vi "Main Tclk.vi"() -> ()   [LabVIEW 2018] (continued)
                        n3304 = call <vilib>:"Flatten Pixmap.vi"("colors"=u32[] [16777222, 65793, 131586, 197379, 263172, 328965, 394758, 460551, 526344, 592137, 657930, 723723, 789516, 855309, 921102, 986895, 1052688, 1118481, 1184274, 1250067, 1315860, 1381653, 1447446, 1513239, 1579032, 1644825, 1710618, 1776411, 1842204, 1907997, 1973790, 2039583, 2105376, 2171169, 2236962, 2302755, 2368548, 2434341, 2500134, 2565927, 2631720, 2697513, 2763306, 2829099, 2894892, 2960685, 3026478, 3092271, 3158064, 3223857, 3289650, 3355443, 3421236, 3487029, 3552822, 3618615, 3684408, 3750201, 3815994, 3881787, 3947580, 4013373, 4079166, 4144959, 4210752, 4276545, 4342338, 4408131, 4473924, 4539717, 4605510, 4671303, 4737096, 4802889, 4868682, 4934475, 5000268, 5066061, 5131854, 5197647, 5263440, 5329233, 5395026, 5460819, 5526612, 5592405, 5658198, 5723991, 5789784, 5855577, 5921370, 5987163, 6052956, 6118749, 6184542, 6250335, 6316128, 6381921, 6447714, 6513507, 6579300, 6645093, 6710886, 6776679, 6842472, 6908265, 6974058, 7039851, 7105644, 7171437, 7237230, 7303023, 7368816, 7434609, 7500402, 7566195, 7631988, 7697781, 7763574, 7829367, 7895160, 7960953, 8026746, 8092539, 8158332, 8224125, 8289918, 8355711, 8421504, 8487297, 8553090, 8618883, 8684676, 8750469, 8816262, 8882055, 8947848, 9013641, 9079434, 9145227, 9211020, 9276813, 9342606, 9408399, 9474192, 9539985, 9605778, 9671571, 9737364, 9803157, 9868950, 9934743, 10000536, 10066329, 10132122, 10197915, 10263708, 10329501, 10395294, 10461087, 10526880, 10592673, 10658466, 10724259, 10790052, 10855845, 10921638, 10987431, 11053224, 11119017, 11184810, 11250603, 11316396, 11382189, 11447982, 11513775, 11579568, 11645361, 11711154, 11776947, 11842740, 11908533, 11974326, 12040119, 12105912, 12171705, 12237498, 12303291, 12369084, 12434877, 12500670, 12566463, 12632256, 12698049, 12763842, 12829635, 12895428, 12961221, 13027014, 13092807, 13158600, 13224393, 13290186, 13355979, 13421772, 13487565, 13553358, 13619151, 13684944, 13750737, 13816530, 13882323, 13948116, 14013909, 14079702, 14145495, 14211288, 14277081, 14342874, 14408667, 14474460, 14540253, 14606046, 14671839, 14737632, 14803425, 14869218, 14935011, 15000804, 15066597, 15132390, 15198183, 15263976, 15329769, 15395562, 15461355, 15527148, 15592941, 15658734, 15724527, 15790320, 15856113, 15921906, 15987699, 16053492, 16119285, 16185078, 16250871, 16316664, 16382457, 16448250, 16514043, 16579836, 16645629, 16711422, 16448250] ("256 gray scale"), "8-bit pixmap"=w9681) -> ("image data"=w9684:T52)  [unwired: 4 in, 5 out]
                        n3305 = call <vilib>:"Write PNG File.vi"("image data"=w9684, "path to PNG file"=w9685) -> ()  [unwired: 1 in, 9 out]
                      }
                    }
                  }
                }
                n3306 = Open/Create/Replace File(file path (use dialog)=w9608) -> (error out=w9610:errorcluster)  [unwired: 5 in, 2 out]
                n3307 = Unbundle By Name(w9610) -> ("status"=w9609:bool)
                n3308 = local read "Recipe input"() -> (w9606:T7)
                n3309 = case shown="False" w9609 {
                  tunnel: w9608 -> [w9663 w9664]
                  tunnel: [w9662 w9664] -> w9611
                  frame False {
                    n3310 = Delete(path (use dialog)=w9663) -> (deleted path=w9662:path)  [unwired: 4 in, 2 out]
                  }
                  frame True {
                  }
                }
                n3311 = call "Recipe read write.vi"("Write"=TRUE, "Recipe path"=w9611, "Write input"=w9606) -> ()  [unwired: 5 in, 4 out]
                n3312 = local read "FIB"() -> (w9602:bool)
                n3313 = Greater Than 0?(x="SEM-FIB Delay (s)") -> (x > 0?=w9600:bool)
                n3314 = Compound Arithmetic op=AND(w9600, "After SEM", w9602) -> (w9604:bool)
                n3315 = case shown="True" w9604 {
                  tunnel: "SEM-FIB Delay (s)" -> [_ w9622]
                  frame False {
                  }
                  frame True {
                    n3316 = local read "FIB blank condenser %"() -> (w9631:u8)
                    n3317 = Number To Decimal String(number=w9622) -> (decimal integer string=w9626:string)  [unwired: 1 in]
                    n3318 = expression code="x*10"(w9622) -> (w9623:u32)
                    n3319 = for {
                      N: w9623 -> [_]
                      stop <- w9634 stop-if-true
                      n3320 = local read "Mill Manual Pause"() -> (w9635:bool)
                      n3321 = local read "FIB"() -> (w9637:bool)
                      n3322 = Wait Until Next ms Multiple(millisecond multiple=u32 100) -> ()  [unwired: 1 out]
                      n3323 = Not(x=w9637) -> (.not. x?=w9636:bool)
                      n3324 = Or(x=w9636, y=w9635) -> (x .or. y?=w9634:bool)
                    }
                    n3325 = Concatenate Strings(w9626, " s delay after SEM..." ("string")) -> (w9624:string)
                    n3326 = Less?(x=w9631, y=u8 100) -> (x < y?=w9633:bool)
                    n3327 = Greater Or Equal?(x=w9622, y=5.0) -> (x >= y?=w9632:bool)
                    n3328 = local write "Status message"(w9624) -> ()
                    n3329 = To Single Precision Float(number=w9631) -> (single precision float=w9630:sgl)
                    n3330 = Compound Arithmetic op=AND(w9633, w9632) -> (w9629:bool)
                    n3331 = case shown="True" w9629 {
                      tunnel: w9630 -> [_ w9640]
                      tunnel: w9622 -> [_ w9639]
                      frame False {
                      }
                      frame True {
                        n3332 = stacked-sequence {
                          seq-local: [w9642 _ _ _] -> [_ w9650 _ _]
                          seq-local: [w9641 _ _ _] -> [_ w9648 _ w9659]
                          seq-local: [_ w9649 _ _] -> [_ _ _ w9660]
                          tunnel: w9640 -> [_ w9647 _ _]
                          tunnel: w9639 -> [_ _ w9653 _]
                          frame #0 {
                            n3333 = local read "Api"() -> (w9644:refnum<k7>)
                            n3334 = call "SmartSEM Remote API get float.vi"("lpszParam"="AP_FIB_CONDENSER" ("Status message"), "ActiveX Container"=w9644) -> ("vValue"=w9641:sgl, "reference out"=w9642:refnum<k7>)  [unwired: 7 in, 1 out]
                          }
                          frame #1 {
                            n3335 = Compound Arithmetic op=MULTIPLY(w9648, w9647, sgl 0.01 ("value")) -> (w9646:sgl)
                            n3336 = call "SmartSEM Remote API set float.vi"("vValue"=w9646, "lpszParam"="AP_FIB_CONDENSER" ("Status message"), "ActiveX Container"=w9650) -> ("reference out"=w9649:refnum<k7>)  [unwired: 7 in, 1 out]
                          }
                          frame #2 {
                            n3337 = expression code="(x-3)*10"(w9653) -> (w9652:u32)
                            n3338 = for {
                              N: w9652 -> [_]
                              stop <- w9654 stop-if-true
                              n3339 = local read "Mill Manual Pause"() -> (w9655:bool)
                              n3340 = local read "FIB"() -> (w9657:bool)
                              n3341 = Wait Until Next ms Multiple(millisecond multiple=u32 100) -> ()  [unwired: 1 out]
                              n3342 = Not(x=w9657) -> (.not. x?=w9656:bool)
                              n3343 = Or(x=w9656, y=w9655) -> (x .or. y?=w9654:bool)
                            }
                          }
                          frame #3 {
                            n3344 = call "SmartSEM Remote API set float.vi"("vValue"=w9659, "lpszParam"="AP_FIB_CONDENSER" ("Status message"), "ActiveX Container"=w9660) -> ()  [unwired: 7 in, 2 out]
                          }
                        }
                      }
                    }
                  }
                }
              }
              frame #40 {
                n3345 = local read "Milling para"() -> (w9706:T35)
                n3346 = local read "SEM Scan Parameters"() -> (w9726:T26)
                n3347 = local read "Temp array"() -> (w9787:sgl[])
                n3348 = local read "Alert Settings"() -> (w9780:T36)
                n3349 = Unbundle By Name(w9706) -> ("FIB PID target"=w9761:sgl, "FIB PID on"=w9766:bool, "FIB PID measured"=w9764:u8)
                n3350 = Unbundle By Name(w9726) -> ("Pixel size (nm)"=w9721:sgl)
                n3351 = Unbundle By Name(w9706) -> ("FIB PID on"=w9728:bool, "FIB PID measured"=w9727:u8, "Lines auto pause"=w9767:u16)
                n3352 = Unbundle By Name(w9780) -> ("Focus index warning"=w9785:bool)
                n3353 = Unbundle By Name(w9706) -> ("Z-step (nm)"=w9768:dbl)
                n3354 = local read "FI below limit counts"() -> (w9786:u8)
                n3355 = Unbundle By Name(w9780) -> ("Focus index stop limit"=w9783:sgl)
                n3356 = Unbundle By Name(w9780) -> ("Temp limit auto"=w9790:bool)
                n3357 = local read "Focus Index"() -> (w9770:sgl)
                n3358 = Array Size(array=w9787) -> (size(s)=w9791:i32)
                n3359 = Equal?(x=u8 3, y=w9764) -> (x = y?=w9765:bool)
                n3360 = In Range and Coerce(upper limit=sgl 50.0, x=w9721, lower limit=sgl 8.0) -> (coerced(x)=w9722:sgl)  [unwired: 1 out]
                n3361 = Greater Or Equal?(x=w9791, y=10 ("x")) -> (x >= y?=w9789:bool)
                n3362 = And(x=w9766, y=w9765) -> (x .and. y?=w9762:bool)
                n3363 = And(x=w9789, y=w9790) -> (x .and. y?=w9788:bool)
                n3364 = Multiply(x=w9767, y=w9768) -> (x*y=w9725:dbl)
                n3365 = case shown="True" w9762 {
                  tunnel: w9761 -> [_ w9805]
                  tunnel: [FALSE w9804] -> w9760
                  frame False {
                  }
                  frame True {
                    n3366 = local read "Faraday Cup (nA)"() -> (w9806:sgl)
                    n3367 = Greater?(x=w9805, y=w9806) -> (0:w9804:bool)
                  }
                }
                "Faraday Cup < Milling current" <- w9760
                n3368 = case shown="True" w9788 {
                  tunnel: w9787 -> [_ w9843]
                  tunnel: w9780 -> [w9837 w9844]
                  tunnel: [w9837 w9838] -> _
                  frame False {
                  }
                  frame True {
                    n3369 = call "Auto limits.vi"("Minimum half range"=0.8, "# of interquartile range or stdev"=4.0 ("# of sigma"), "Input array"=w9843) -> ("Low limit"=w9841:dbl, "High limit"=w9842:dbl)  [unwired: 6 in, 1 out]
                    n3370 = Bundle By Name(cluster=w9844, "High limit (F)"=w9842, "Low limit (F)"=w9841) -> (w9838:T36)
                    n3371 = local write "Alert Settings"(w9838) -> ()
                  }
                }
                n3372 = Divide(x=w9722, y=w9725) -> (x/y=w9707:dbl)
                n3373 = Greater Or Equal?(x=w9770, y=w9783) -> (x >= y?=w9784:bool)
                n3374 = case shown="True" w9728 {
                  tunnel: [FALSE w9809] -> w9777
                  tunnel: w9727 -> [_ w9808]
                  frame False {
                  }
                  frame True {
                    n3375 = case shown="3" w9808 {
                      tunnel: [w9811 w9816 w9820 w9827 FALSE] -> w9809
                      frame 0 {
                        n3376 = local read "Specimen I out of bound"() -> (w9814:bool)
                        n3377 = local read "BD1 out of bound"() -> (w9810:bool)
                        n3378 = local read "BD2 out of bound"() -> (w9813:bool)
                        n3379 = local read "Milling I out of bound"() -> (w9812:bool)
                        n3380 = Compound Arithmetic op=OR(w9814, w9810, w9813, w9812) -> (w9811:bool)
                      }
                      frame 1 {
                        n3381 = local read "Specimen I out of bound"() -> (w9818:bool)
                        n3382 = local read "BD1 out of bound"() -> (w9815:bool)
                        n3383 = local read "BD2 out of bound"() -> (w9817:bool)
                        n3384 = Compound Arithmetic op=OR(w9818, w9815, w9817) -> (w9816:bool)
                      }
                      frame 2 {
                        n3385 = local read "Specimen I out of bound"() -> (w9823:bool)
                        n3386 = local read "BD1 out of bound"() -> (w9819:bool)
                        n3387 = local read "BD2 out of bound"() -> (w9822:bool)
                        n3388 = local read "Milling I out of bound"() -> (w9821:bool)
                        n3389 = Compound Arithmetic op=OR(w9823, w9819, w9822, w9821) -> (w9820:bool)
                      }
                      frame 3 {
                        n3390 = local read "Specimen I out of bound"() -> (w9826:bool)
                        n3391 = local read "BD2 out of bound"() -> (w9825:bool)
                        n3392 = local read "Milling I out of bound"() -> (w9828:bool)
                        n3393 = And(x=w9826, y=w9825) -> (x .and. y?=w9824:bool)
                        n3394 = Compound Arithmetic op=OR(w9824, w9828) -> (w9827:bool)
                      }
                      frame 100, Default {
                      }
                    }
                  }
                }
                n3395 = Round Toward +Infinity(x=w9707) -> (ceil(x): smallest int >= x=w9708:dbl)
                n3396 = Greater Or Equal?(x=sgl 1e-06, y=w9770) -> (x >= y?=w9729:bool)
                n3397 = To Unsigned Byte Integer(number=w9708) -> (unsigned 8bit integer=w9723:u8)
                n3398 = case shown="False" w9784 {
                  tunnel: w9786 -> [w9835 _]
                  tunnel: w9729 -> [w9833 _]
                  tunnel: [w9830 w9836] -> w9709
                  frame False {
                    n3399 = Select(t=u8 2 ("FI below limit counts"), s=w9833, f=u8 1 ("FI below limit counts")) -> (s? t:f=w9834:u8)
                    n3400 = Add(x=w9835, y=w9834) -> (x+y=w9830:u8)
                    n3401 = local write "FI below limit counts"(w9830) -> ()
                  }
                  frame True {
                    w9836 = u8 0 ("FI below limit counts")
                    n3402 = local write "FI below limit counts"(w9836) -> ()
                  }
                }
                n3403 = Less Or Equal?(x=w9723, y=w9709) -> (x <= y?=w9730:bool)
                n3404 = And(x=w9785, y=w9730) -> (x .and. y?=→"Focus index stop trigger active":bool)
                n3405 = Multiply(x=w9723, y=w9725) -> (x*y=→"Z removal stop threshold Z(nm)":dbl)
                n3406 = local read "FIB CL I out of bound counts"() -> (w9710:u8)
                n3407 = local read "Milling para"() -> (w9716:T35)
                n3408 = local read "Est. cycle time (s)"() -> (w9736:u32)
                n3409 = local read "SEM Specimen I array"() -> (w9757:sgl[])
                n3410 = local read "SEM Specimen I"() -> (w9751:dbl)
                n3411 = local read "Alert Settings"() -> (w9705:T36)
                n3412 = local read "Beam Dump 1 (nA)"() -> (w9781:sgl)
                n3413 = local read "Faraday Cup (nA)"() -> (w9775:sgl)
                n3414 = local read "Milling Z voltage array"() -> (w9759:sgl[])
                n3415 = local read "Auto re-engage"() -> (w9754:bool)
                n3416 = Unbundle By Name(w9705) -> ("Milling Z voltage alarm"=w9740:bool)
                n3417 = local read "FIB"() -> (w9741:bool)
                n3418 = Unbundle By Name(w9716) -> ("Line milling time (s)"=w9715:sgl, "Lines auto pause"=w9714:u16)
                n3419 = Not(x=w9754) -> (.not. x?=w9753:bool)
                n3420 = local read "SEM Specimen I low limit array"() -> (w9750:sgl[])
                n3421 = expression code="abs(x*0.05)"(w9775) -> (w9734:sgl)
                n3422 = local read "SEM Specimen I high limit array"() -> (w9747:sgl[])
                n3423 = expression code="21600/x"(w9736) -> (w9735:u32)
                n3424 = Compound Arithmetic op=AND(w9753, w9741, w9740) -> (w9752:bool)
                n3425 = Increment(x=w9710) -> (x+1=w9778:u8)
                n3426 = call "Auto limits.vi"("Minimum half range"=0.1, "# of interquartile range or stdev"=4.0 ("# of sigma"), "Length"=w9735, "Input array"=w9757) -> ("Low limit"=w9749:dbl, "High limit"=w9746:dbl)  [unwired: 5 in, 1 out]
                n3427 = Unbundle By Name(w9705) -> ("Specimen @ SEM alarm"=w9737:bool)
                n3428 = Select(t=w9778, s=w9777, f=u8 0 ("y")) -> (s? t:f=w9717:u8)
                n3429 = case shown="True" w9752 {
                  tunnel: w9759 -> [_ w9801]
                  tunnel: [FALSE w9794] -> w9755
                  frame False {
                  }
                  frame True {
                    n3430 = local read "Milling Z voltage (V)"() -> (w9797:sgl)
                    n3431 = call "Auto limits.vi"("Minimum half range"=0.05, "# of interquartile range or stdev"=1.0 ("# of sigma"), "Length"=10, "Input array"=w9801) -> ("Low limit"=w9796:dbl, "High limit"=w9795:dbl)  [unwired: 5 in, 1 out]
                    n3432 = In Range and Coerce(upper limit=w9795, x=w9797, lower limit=w9796) -> (In Range?=w9798:bool)  [unwired: 1 out]
                    n3433 = Not(x=w9798) -> (.not. x?=w9794:bool)
                  }
                }
                "Milling Z voltage spike" <- w9755
                n3434 = Multiply(x=w9715, y=w9714) -> (x*y=w9713:sgl)
                n3435 = To Single Precision Float(number=w9746) -> (single precision float=w9744:sgl)
                n3436 = To Single Precision Float(number=w9749) -> (single precision float=w9743:sgl)
                n3437 = In Range and Coerce(upper limit=sgl 1.0, x=w9734, lower limit=sgl 0.0) -> (coerced(x)=w9731:sgl)  [unwired: 1 out]
                n3438 = local write "FIB CL I out of bound counts"(w9717) -> ()
                n3439 = Greater?(x=w9713, y=sgl 6.0) -> (0:w9711:bool)
                n3440 = Less Or Equal?(x=w9781, y=w9731) -> (x <= y?=w9773:bool)
                n3441 = Less Or Equal?(x=w9775, y=sgl 0.1) -> (x <= y?=w9772:bool)
                n3442 = Build Array (concatenate)(w9750, w9743) -> (w9748:sgl[])
                n3443 = Build Array (concatenate)(w9747, w9744) -> (w9745:sgl[])
                n3444 = Or(x=w9773, y=w9772) -> (x .or. y?=→"Beam dump at zero":bool)
                n3445 = Select(t=w9717, s=w9711, f=w9710) -> (s? t:f=w9718:u8)
                n3446 = In Range and Coerce(upper limit=w9744, x=w9751, lower limit=w9743) -> (In Range?=w9756:bool)  [unwired: 1 out]
                n3447 = Greater Or Equal?(x=w9718, y=w9723) -> (x >= y?=→"FIB CL I alarm active":bool)
                n3448 = local write "SEM Specimen I high limit array"(w9745) -> ()
                n3449 = local write "SEM Specimen I low limit array"(w9748) -> ()
                n3450 = Not(x=w9756) -> (.not. x?=w9739:bool)
                n3451 = And(x=w9739, y=w9737) -> (x .and. y?=→"SEM Spec. I spike":bool)
              }
              frame #41 {
                n3452 = local read "Total\nprogress"() -> (w9886:u8)
                n3453 = local read "Milling para"() -> (w9876:T35)
                n3454 = local read "FIB"() -> (w9855:bool)
                n3455 = local read "Alert Settings"() -> (w9856:T36)
                n3456 = Unbundle By Name(w9856) -> ("FIB emission warning"=w9854:bool)
                n3457 = local read "Alert Settings"() -> (w9864:T36)
                n3458 = local read "SW error warning active"() -> (w9862:bool)
                n3459 = Equal?(x=w9886, y=u8 100) -> (x = y?=w9885:bool)
                n3460 = And(x=w9855, y=w9854) -> (x .and. y?=w9853:bool)
                n3461 = local read "Temp gradient (F/min)"() -> (w9852:dbl)
                n3462 = Unbundle By Name(w9856) -> ("High limit (F)"=w9880:sgl, "Low limit (F)"=w9879:sgl, "Pause 3D-ING"=w9877:bool)
                n3463 = Unbundle By Name(w9864) -> ("SW error warning"=w9863:bool)
                n3464 = case shown="True" w9885 {
                  tunnel: [w9986 FALSE ("Initialization")] -> w9882
                  frame False {
                    n3465 = local read "Machine Type"() -> (w9985:u8)
                    n3466 = case shown="0, Default" w9985 {
                      tunnel: [w9989 w10001] -> w9986
                      frame 0, Default {
                        n3467 = local read "Hardware Configuration"() -> (w9988:T25)
                        n3468 = Unbundle By Name(w9988) -> ("Eanable COM"=w9987:bool)
                        n3469 = case shown="True" w9987 {
                          tunnel: [FALSE w9997] -> w9989
                          frame False {
                          }
                          frame True {
                            w9995 = TRUE ("Initialization")
                            n3470 = local read "COM port"() -> (w9996:refnum<visa-resource-name>)
                            n3471 = call "Remcon32 command.vi"("Close session"=w9995, "Initialization"=w9995, "SEM command"="eht?", "COM port in"=w9996) -> ("SEM reply"=w9993:string)  [unwired: 4 in, 3 out]
                            n3472 = Fract/Exp String To Number(string=w9993, default (0 dbl)=sgl 0.0 ("value (0)")) -> (number=w9991:sgl)  [unwired: 3 out]
                            n3473 = Equal To 0?(x=w9991) -> (x = 0?=w9997:bool)
                            "EHT off" <- w9997
                          }
                        }
                      }
                      frame 2 {
                        n3474 = local read "Api"() -> (w9998:refnum<k7>)
                        n3475 = call "SmartSEM Remote API get float.vi"("lpszParam"="AP_ACTUALKV", "ActiveX Container"=w9998) -> ("vValue"=w10000:sgl)  [unwired: 7 in, 2 out]
                        n3476 = Equal To 0?(x=w10000) -> (x = 0?=w10001:bool)
                        n3477 = local write "EHT off"(w10001) -> ()
                      }
                    }
                  }
                  frame True {
                    w10006 = FALSE ("FIB")
                    n3478 = local write "FIB"(w10006) -> ()
                    n3479 = local write "3D FIB-SEM"(w10006) -> ()
                    n3480 = local write "Mill Stop"(TRUE ("Initialization")) -> ()
                    n3481 = local read "WatchDog Mode"() -> (w10002:u16)
                    n3482 = local read "Machine Type"() -> (w10008:u8)
                    n3483 = local write "Status message"("3D FIB-SEM Completed" ("Status message")) -> ()
                    n3484 = call "FM Gen Pulse for FIB-SEM.vi"("WatchDog Mode"=w10002, "State Value"=i16 7) -> ()  [unwired: 7 in, 3 out]
                    n3485 = case shown="1" w10008 {
                      frame 0, Default {
                      }
                      frame 1 {
                        n3486 = stacked-sequence {
                          frame #0 {
                            w10010 = FALSE ("Mill")
                            n3487 = local write "Mill"(w10010) -> ()
                            n3488 = local write "Mill Stop"(TRUE ("Rect Milling Stop")) -> ()
                            n3489 = local write "Mill Manual Pause"(w10010) -> ()
                          }
                          frame #1 {
                            w10012 = TRUE ("Initialization")
                            n3490 = local read "COM port"() -> (w10018:refnum<visa-resource-name>)
                            n3491 = call "FIB mode.vi"("Initialization"=w10012, "FIB mode"=T10."SEM", "COM port in"=w10018) -> ("COM port out"=w10017:refnum<visa-resource-name>)  [unwired: 7 in, 1 out]
                            n3492 = call "Remcon32 command.vi"("SEM command"="edx 0", "COM port in"=w10017) -> ("COM port out"=w10016:refnum<visa-resource-name>)  [unwired: 6 in, 3 out]
                            n3493 = call "Remcon32 command.vi"("Close session"=w10012, "SEM command"="frez", "COM port in"=w10016) -> ()  [unwired: 5 in, 4 out]
                          }
                        }
                      }
                      frame 2 {
                        n3494 = local read "Api"() -> (w10023:refnum<k7>)
                        n3495 = call "SmartSEM Remote API FIB mode.vi"("FIB mode"=T50."SEM", "ActiveX Container"=w10023) -> ("error out"=w10019:errorcluster, "reference out"=w10020:refnum<k7>)  [unwired: 8 in]
                        n3496 = invoke class="_EMApi" method="Execute"(reference=w10020, error in=w10019, "lpszCommand"="CMD_FREEZE_ALL") -> ()  [unwired: 1 in, 4 out]
                      }
                    }
                    n3497 = local read "Email recipents file"() -> (w10004:path)
                    n3498 = Delete(path (use dialog)=w10004) -> ()  [unwired: 4 in, 3 out]
                  }
                }
                n3499 = case shown="True" w9853 {
                  tunnel: [FALSE w9942] -> w9865
                  tunnel: w9876 -> [_ w9961]
                  frame False {
                  }
                  frame True {
                    w9941 = u8 0 ("f")
                    n3500 = local read "FIB emission below limit counts"() -> (w9952:u8)
                    n3501 = local read "FIB suppressor below limit counts"() -> (w9946:u8)
                    n3502 = Unbundle By Name(w9961) -> ("Suppressor (V)"=w9954:sgl, "Emission (uA)"=w9955:dbl)
                    n3503 = local read "Machine Type"() -> (w9962:u8)
                    n3504 = local read "Alert Settings"() -> (w9966:T36)
                    n3505 = case shown="2" w9962 {
                      tunnel: [w9971 w9975 w9983] -> w9963
                      tunnel: w9955 -> [w9969 w9976 w9982]
                      tunnel: [w9970 w9974 w9979] -> w9951
                      tunnel: w9954 -> [_ _ w9980]
                      tunnel: [FALSE FALSE w9978] -> w9947
                      frame 0, Default {
                        n3506 = local read "HV Data Output"() -> (w9972:T18)
                        n3507 = Unbundle By Name(w9972) -> ("Emission (uA)"=w9971:sgl)
                        n3508 = Greater Or Equal?(x=w9969, y=w9971) -> (x >= y?=w9970:bool)
                      }
                      frame 1 {
                        n3509 = local read "FIB Parameters"() -> (w9977:T19)
                        n3510 = Unbundle By Name(w9977) -> ("FIB emission (uA)"=w9975:sgl)
                        n3511 = Greater Or Equal?(x=w9976, y=w9975) -> (x >= y?=w9974:bool)
                      }
                      frame 2 {
                        n3512 = local read "Capella HV Data Output"() -> (w9984:T17)
                        n3513 = Unbundle By Name(w9984) -> ("Suppressor (V)"=w9981:sgl, "Emission Actual (uA)"=w9983:sgl)
                        n3514 = Greater Or Equal?(x=w9982, y=w9983) -> (x >= y?=w9979:bool)
                        n3515 = Greater Or Equal?(x=w9980, y=w9981) -> (x >= y?=w9978:bool)
                      }
                    }
                    n3516 = Unbundle By Name(w9966) -> ("High limit"=w9965:dbl, "Low limit"=w9964:dbl)
                    n3517 = In Range and Coerce(upper limit=w9965, x=w9963, lower limit=w9964) -> (In Range?=w9940:bool)  [unwired: 1 out]
                    n3518 = Increment(x=w9952) -> (x+1=w9953:u8)
                    n3519 = Increment(x=w9946) -> (x+1=w9948:u8)
                    n3520 = Not(x=w9940) -> (.not. x?=→"FIB emission limit warning active":bool)
                    n3521 = Select(t=w9953, s=w9951, f=w9941) -> (s? t:f=w9950:u8)
                    n3522 = Select(t=w9948, s=w9947, f=w9941) -> (s? t:f=w9949:u8)
                    n3523 = local write "FIB emission limit warning armed"(w9940) -> ()
                    n3524 = local write "FIB emission below limit counts"(w9950) -> ()
                    n3525 = local write "FIB suppressor below limit counts"(w9949) -> ()
                    n3526 = local read "Est. cycle time (s)"() -> (w9959:u32)
                    n3527 = Quotient & Remainder(x=u32 300, y=w9959) -> (floor(x/y)=w9958:u32)  [unwired: 1 out]
                    n3528 = In Range and Coerce(upper limit=u32 10, x=w9958, lower limit=u32 2 ("x")) -> (coerced(x)=w9945:u32)  [unwired: 1 out]
                    n3529 = Greater Or Equal?(x=w9952, y=w9945) -> (x >= y?=w9943:bool)
                    n3530 = Greater Or Equal?(x=w9946, y=w9945) -> (x >= y?=w9944:bool)
                    n3531 = Or(x=w9943, y=w9944) -> (x .or. y?=w9942:bool)
                  }
                }
                n3532 = local read "Temp (F)"() -> (w9881:sgl)
                n3533 = Absolute Value(x=w9852) -> (abs(x)=w9849:dbl)
                n3534 = And(x=w9863, y=w9862) -> (x .and. y?=w9861:bool)
                n3535 = Greater Or Equal?(x=w9849, y=0.2) -> (x >= y?=w9851:bool)
                n3536 = In Range and Coerce(upper limit=w9880, x=w9881, lower limit=w9879) -> (In Range?=w9848:bool)  [unwired: 1 out]
                "Temperature recovery active" <- w9848
                n3537 = Not(x=w9848) -> (.not. x?=w9847:bool)
                n3538 = And(x=w9851, y=w9847) -> (x .and. y?=w9846:bool)
                "Temperature warning active" <- w9846
                n3539 = local read "Faraday Cup < Milling current"() -> (w9867:bool)
                n3540 = And(x=w9846, y=w9877) -> (x .and. y?=w9878:bool)
                n3541 = local read "Focus index stop trigger active"() -> (w9875:bool)
                n3542 = local read "FIB CL I alarm active"() -> (w9869:bool)
                n3543 = local read "Alert Settings"() -> (w9874:T36)
                n3544 = local read "Beam dump at zero"() -> (w9871:bool)
                n3545 = Unbundle By Name(w9874) -> ("FIB CL current alarm"=w9870:bool, "Beam Dump 1 alarm"=w9872:bool)
                n3546 = local read "Milling Z voltage spike"() -> (w9866:bool)
                n3547 = local read "SEM Spec. I spike"() -> (w9868:bool)
                n3548 = local read "API timeout"() -> (w9845:bool)
                n3549 = And(x=w9869, y=w9870) -> (x .and. y?=w9859:bool)
                n3550 = And(x=w9872, y=w9871) -> (x .and. y?=w9873:bool)
                n3551 = Compound Arithmetic op=OR(w9882, w9865, w9878, w9875, w9859, w9873, w9868, w9867, w9866, w9861, w9845) -> (w9883:bool)
                n3552 = local read "Machine Type"() -> (w9857:u8)
                n3553 = case shown="0, Default" w9857 {
                  tunnel: [w9887 FALSE FALSE] -> w9860
                  frame 0, Default {
                    n3554 = local read "HV Data Output"() -> (w9892:T18)
                    n3555 = Unbundle By Name(w9892) -> ("Suppressor (V)"=w9891:sgl)
                    n3556 = local read "Faraday cup I low"() -> (w9888:bool)
                    n3557 = Greater Or Equal?(x=sgl -1800.0, y=w9891) -> (x >= y?=w9889:bool)
                    n3558 = Or(x=w9889, y=w9888) -> (x .or. y?=w9887:bool)
                  }
                  frame 1 {
                  }
                  frame 2 {
                  }
                }
                n3559 = And(x=w9859, y=w9860) -> (x .and. y?=w9858:bool)
                n3560 = case shown="True" w9883 {
                  tunnel: w9865 -> [_ w9912]
                  tunnel: w9858 -> [_ w9913]
                  frame False {
                    n3561 = local read "Milling Z voltage (V)"() -> (→"Last good milling Z voltage (V)":sgl)
                  }
                  frame True {
                    w9914 = TRUE ("Rect Mill Manual Pause")
                    n3562 = Or(x=w9912, y=w9913) -> (x .or. y?=w9911:bool)
                    n3563 = local read "Last good FI"() -> (w9928:sgl)
                    n3564 = local read "Hardware Configuration"() -> (w9902:T25)
                    n3565 = local read "Milling para"() -> (w9916:T35)
                    n3566 = local read "SEM Scan Parameters"() -> (w9926:T26)
                    n3567 = shared-variable ".\\Zeiss Library.lvlib\\Timestamp"() -> (w9931:timestamp)  [unwired: 1 in, 1 out]
                    n3568 = local read "FIB slice #"() -> (w9897:u32)
                    n3569 = Unbundle By Name(w9902) -> ("Shutter Drive"=w9903:tag)
                    n3570 = local write "Pause for reheat"(w9914) -> ()
                    n3571 = local write "3D image paused active"(w9914) -> ()
                    n3572 = local write "Mill Manual Pause"(w9914) -> ()
                    n3573 = local read "Damping"() -> (w9908:bool)
                    n3574 = local read "Re-engage Files"() -> (w9917:path)
                    n3575 = Unbundle By Name(w9916) -> ("Auto reheat"=w9909:bool, "FIB PID target"=w9915:sgl)
                    n3576 = Equal To 0?(x=w9897) -> (x = 0?=w9896:bool)
                    n3577 = local write "Pre-reheat FI"(w9928) -> ()
                    n3578 = local write "Config Tabs"(T24."FIB Milling" ("Config Tabs")) -> ()
                    n3579 = local write "Pre-reheat time"(w9931) -> ()
                    n3580 = case shown="True" w9896 {
                      frame False {
                      }
                      frame True {
                        n3581 = local read "Milling Z voltage (V)"() -> (w9933:sgl)
                        n3582 = local write "Last good milling Z voltage (V)"(w9933) -> ()
                      }
                    }
                    n3583 = call "Shutter Swing V3.vi"("Shutter Drive"=w9903, "Damping"=w9908, "Shutter close"=TRUE) -> ("Shutter close fdbk"=w9907:bool, "Fail #"=w9906:u8, "SEM shutter status"=w9905:string, "Color Box"=w9904:u32)  [unwired: 2 in, 3 out]
                    n3584 = Unbundle By Name(w9926) -> ("X center (um)"=w9929:sgl, "Y center (um)"=w9930:sgl, "Y stig"=w9924:sgl[][])
                    n3585 = property on="SEM shutter status" class="Str"("Text.BGColor"=w9904) -> ()  [unwired: 2 in, 2 out]
                    n3586 = local write "SEM shutter status"(w9905) -> ()
                    n3587 = local write "Fail #"(w9906) -> ()
                    n3588 = local write "SEM Shutter"(w9907) -> ()
                    n3589 = And(x=w9911, y=w9909) -> (x .and. y?=w9925:bool)
                    n3590 = Build Path(base path=w9917, name or relative path="pre.png " ("command line")) -> (appended path=w9922:path)
                    n3591 = local read "Additional Info"() -> (w9900:cluster{"Restart flag":u8, "Stage move flag":u8})
                    n3592 = local read "3D FIB-SEM Files"() -> (w9920:path)
                    n3593 = local write "Pre-reheat X center (um)"(w9929) -> ()
                    n3594 = local write "Pre-reheat Y center (um)"(w9930) -> ()
                    n3595 = local write "Pre-reheat Y stig"(w9924) -> ()
                    n3596 = Bundle By Name(cluster=w9900, "Restart flag"=u8 10) -> (w9899:cluster{"Restart flag":u8, "Stage move flag":u8})
                    n3597 = local write "Status message"("Paused" ("Status message")) -> ()
                    n3598 = case shown="True" w9925 {
                      tunnel: w9915 -> [_ w9934]
                      frame False {
                      }
                      frame True {
                        w9938 = TRUE ("Request to reheat")
                        n3599 = local read "Reheat Output"() -> (w9937:T21)
                        n3600 = local write "Start Reheat"(w9938) -> ()
                        n3601 = Bundle By Name(cluster=w9937, "Reheat Success"=FALSE) -> (w9936:T21)
                        n3602 = local write "Reheat Output"(w9936) -> ()
                        "Auto reheat running" <- w9938
                        "Pre-reheat FIB PID target" <- w9934
                      }
                    }
                    n3603 = local write "Additional Info"(w9899) -> ()
                    n3604 = Build Path(base path=w9920, name or relative path="LG low res.png " ("command line")) -> (appended path=w9921:path)
                    n3605 = property on="Mill Manual Pause" class="Bool (strict)"("DisabledEnum"=T44."Disabled and Grayed Out" ("Disabled")) -> ()  [unwired: 2 in, 2 out]
                    n3606 = Copy(9:TRUE ("run minimized? (F)"), 10:w9922, 11:w9921) -> ()  [unwired: 2 in, 3 out]
                  }
                }
              }
              frame #42 {
                w10063 = FALSE ("Rect Milling Line Paused")
                w10056 = TRUE ("Rect Milling Resume")
                n3607 = local read "FIB"() -> (w10058:bool)
                n3608 = local read "Initial Options"() -> (w10059:T27)
                n3609 = local read "FIB HW Config"() -> (w10062:T23)
                n3610 = shared-variable "My Computer\\Zeiss Library.lvlib\\Milling Resume"(w10056) -> ()  [unwired: 1 in, 1 out]
                n3611 = shared-variable "My Computer\\Zeiss Library.lvlib\\Milling Line Paused"(w10063) -> ()  [unwired: 1 in, 1 out]
                n3612 = local write "Reset Focus"(w10063) -> ()
                n3613 = case shown="True" w10058 {
                  frame False {
                    n3614 = local read "Machine Type"() -> (w10084:u8)
                    n3615 = local write "Mill"(FALSE ("Mill")) -> ()
                    n3616 = local write "Mill Stop"(TRUE ("Rect Milling Stop")) -> ()
                    n3617 = local read "Hardware Configuration"() -> (w10075:T25)
                    n3618 = case shown="2" w10084 {
                      frame 0, Default {
                      }
                      frame 1 {
                        n3619 = stacked-sequence {
                          frame #0 {
                            n3620 = Wait (ms)(milliseconds to wait=u32 1000) -> ()  [unwired: 1 out]
                          }
                          frame #1 {
                            w10086 = TRUE ("Initialization")
                            n3621 = local read "COM port"() -> (w10092:refnum<visa-resource-name>)
                            n3622 = call "FIB mode.vi"("Initialization"=w10086, "FIB mode"=T10."SEM", "COM port in"=w10092) -> ("COM port out"=w10091:refnum<visa-resource-name>)  [unwired: 7 in, 1 out]
                            n3623 = call "Remcon32 command.vi"("SEM command"="edx 0", "COM port in"=w10091) -> ("COM port out"=w10090:refnum<visa-resource-name>)  [unwired: 6 in, 3 out]
                            n3624 = call "Remcon32 command.vi"("Close session"=w10086, "SEM command"="frez", "COM port in"=w10090) -> ()  [unwired: 5 in, 4 out]
                          }
                        }
                      }
                      frame 2 {
                        n3625 = local read "Api"() -> (w10097:refnum<k7>)
                        n3626 = call "SmartSEM Remote API FIB mode.vi"("FIB mode"=T50."SEM", "ActiveX Container"=w10097) -> ("error out"=w10093:errorcluster, "reference out"=w10094:refnum<k7>)  [unwired: 8 in]
                        n3627 = invoke class="_EMApi" method="Execute"(reference=w10094, error in=w10093, "lpszCommand"="CMD_FREEZE_ALL") -> ()  [unwired: 1 in, 4 out]
                      }
                    }
                    n3628 = Unbundle By Name(w10075) -> ("Shutter Drive"=w10081:tag)
                    n3629 = local read "Damping"() -> (w10074:bool)
                    n3630 = call "Shutter Swing V3.vi"("Shutter Drive"=w10081, "Damping"=w10074, "Shutter close"=FALSE) -> ("Shutter close fdbk"=w10080:bool, "Fail #"=w10077:u8, "SEM shutter status"=w10076:string)  [unwired: 2 in, 4 out]
                    n3631 = Greater Than 0?(x=w10077) -> (x > 0?=w10079:bool)
                    n3632 = local write "SEM shutter status"(w10076) -> ()
                    n3633 = local write "Fail #"(w10077) -> ()
                    n3634 = local write "SEM shutter failed active"(w10079) -> ()
                    n3635 = local write "SEM Shutter"(w10080) -> ()
                  }
                  frame True {
                    n3636 = local read "Mill Stop"() -> (w10099:bool)
                    n3637 = local read "FIB slice #"() -> (w10100:u32)
                    n3638 = case shown="True" w10099 {
                      tunnel: w10100 -> [w10114 w10116]
                      tunnel: [w10113 w10116] -> w10098
                      frame False {
                        n3639 = Increment(x=w10114) -> (x+1=w10113:u32)
                      }
                      frame True {
                        n3640 = local write "FIB"(FALSE ("FIB")) -> ()
                      }
                    }
                    n3641 = local read "Last good milling Z voltage (V)"() -> (w10103:sgl)
                    n3642 = local read "Last milling snapshot"() -> (w10106:path)
                    n3643 = shared-variable ".\\Zeiss Library.lvlib\\Timestamp"() -> (w10109:timestamp)  [unwired: 1 in, 1 out]
                    n3644 = local write "FIB slice #"(w10098) -> ()
                    n3645 = local read "Pause for reheat"() -> (w10110:bool)
                    n3646 = local read "Last good FI"() -> (w10112:sgl)
                    n3647 = local read "Focus Index"() -> (w10111:sgl)
                    n3648 = local read "Hardware Configuration"() -> (w10104:T25)
                    n3649 = local read "Remaining X shift frames"() -> (w10102:u32)
                    n3650 = local read "Remaining Y shift frames"() -> (w10101:u32)
                    n3651 = Unbundle By Name(w10104) -> ("SEM Max FOV (um)"=w10105:sgl)
                    n3652 = Bundle("Timestamp"=w10109, "Last good milling Z voltage (V)"=w10103, "FIB slice #"=w10098, "Pause for reheat"=w10110, "Last good FI"=w10112, "Focus Index"=w10111, "SEM Max FOV (um)"=w10105, "Remaining X shift frames"=w10102, "Remaining Y shift frames"=w10101) -> (w10107:T76)  [unwired: 1 in]
                    n3653 = Flatten To XML(anything=w10107) -> (xml string=w10108:string)
                    n3654 = call-poly <vilib>:"Write to XML File.vi"("XML Input"=w10108, "XML File Path"=w10106) -> ()  [unwired: 7 in, 3 out]
                  }
                }
                n3655 = Unbundle By Name(w10062) -> ("FIB Ext Scan"=w10060:tag)
                n3656 = local write "SEM Options"(w10059) -> ()
                n3657 = call "FIB ext scan.vi"("Ext on"=FALSE ("data"), "FIB Ext Scan"=w10060) -> ()  [unwired: 9 in, 1 out]
                n3658 = local read "Milling para"() -> (w10027:T35)
                n3659 = Bundle By Name(cluster=w10027, "FIB PID reset"=w10056) -> (w10057:T35)
                n3660 = shared-variable ".\\Zeiss Library.lvlib\\FIB PID reset"(w10056) -> ()  [unwired: 1 in, 1 out]
                n3661 = Unbundle By Name(w10027) -> ("FIB PID measured"=w10024:u8, "FIB PID target"=w10025:sgl)
                n3662 = local read "Specimen I (nA)"() -> (w10026:sgl)
                n3663 = local write "Milling para"(w10057) -> ()
                n3664 = case shown="0, Default" w10024 {
                  tunnel: w10026 -> [_ w10073]
                  tunnel: w10025 -> [_ w10069]
                  frame 0, Default {
                    n3665 = local read "Milling I (nA)"() -> (w10064:sgl)
                    n3666 = local write "FIB mill target by spec. I (nA)"(w10064) -> ()
                  }
                  frame 4 {
                    n3667 = Subtract(x=w10069, y=w10073) -> (x-y=w10072:sgl)
                    n3668 = Sign(1:w10069) -> (0:w10068:sgl)
                    n3669 = Sign(1:w10072) -> (0:w10071:sgl)
                    n3670 = Compound Arithmetic op=MULTIPLY(sgl 0.01 ("x"), w10068, w10071) -> (w10067:sgl)
                    n3671 = Add(x=w10067, y="FIB mill target by spec. I (nA)") -> (x+y=w10065:sgl)
                    n3672 = local write "FIB mill target by spec. I (nA)"(w10065) -> ()
                  }
                }
                n3673 = local read "SEM Scan Parameters"() -> (w10043:T26)
                n3674 = local read "WD Stig Aln tile offsets"() -> (w10037:T3)
                n3675 = Unbundle By Name(w10043) -> ("WD (mm)"=w10047:sgl[][], "X stig"=w10049:sgl[][], "Y stig"=w10052:sgl[][], "X aln"=w10053:sgl[][], "Y aln"=w10055:sgl[][], "dX (um)"=w10035:sgl[], "dY (um)"=w10030:sgl[], "Y tiles"=w10044:u8, "X tiles"=w10045:u8)
                n3676 = expression code="(x-1)/2"(w10044) -> (w10032:u8)
                n3677 = expression code="(x-1)/2"(w10045) -> (w10029:u8)
                n3678 = Index Array(array=w10047, index (row)=w10032, index (col)=w10029) -> (element=w10046:sgl)
                n3679 = Index Array(array=w10049, index (row)=w10032, index (col)=w10029) -> (element=w10048:sgl)
                n3680 = Index Array(array=w10052, index (row)=w10032, index (col)=w10029) -> (element=w10051:sgl)
                n3681 = Index Array(array=w10053, index (row)=w10032, index (col)=w10029) -> (element=w10050:sgl)
                n3682 = Index Array(array=w10055, index (row)=w10032, index (col)=w10029) -> (element=w10054:sgl)
                n3683 = Index Array(array=w10035, index=w10032) -> (element=w10034:sgl)
                n3684 = Index Array(array=w10030, index=w10029) -> (element=w10031:sgl)
                n3685 = Subtract(x=w10047, y=w10046) -> (x-y=w10042:sgl[][])
                n3686 = Subtract(x=w10049, y=w10048) -> (x-y=w10041:sgl[][])
                n3687 = Subtract(x=w10052, y=w10051) -> (x-y=w10040:sgl[][])
                n3688 = Subtract(x=w10053, y=w10050) -> (x-y=w10039:sgl[][])
                n3689 = Subtract(x=w10055, y=w10054) -> (x-y=w10038:sgl[][])
                n3690 = Subtract(x=w10035, y=w10034) -> (x-y=w10033:sgl[])
                n3691 = Subtract(x=w10030, y=w10031) -> (x-y=w10028:sgl[])
                n3692 = Bundle By Name(cluster=w10037, "dWD"=w10042, "dX stig"=w10041, "dY stig"=w10040, "dX aln"=w10039, "dY aln"=w10038, "dX (um)"=w10033, "dY (um)"=w10028) -> (w10036:T3)
                n3693 = local write "WD Stig Aln tile offsets"(w10036) -> ()
              }
            }
          }
        }
        n3694 = Wait Until Next ms Multiple(millisecond multiple=u32 100) -> ()  [unwired: 1 out]
      }
      n3695 = while {
        shift-right: [w2816] -> _
        shift-left: _ -> [w2815]
        shift-right: [w2791] -> _
        shift-left: _ -> [w2792]
        shift-right: [w2785] -> _
        shift-left: _ -> [w2784]
        shift-right: [w2774] -> _
        shift-left: _ -> [w2777]
        stop <- "Stop" stop-if-true
        w2722 = sgl 5.0 ("y")
        w2727 = sgl 5.0 ("y")
        n3696 = local read "SEM Status"() -> (w2808:T12)
        n3697 = shared-variable ".\\Zeiss Library.lvlib\\SEMInfo"() -> (w2816:variant)  [unwired: 2 out]
        n3698 = shared-variable ".\\Zeiss Library.lvlib\\Det A Img"() -> (w2791:i16[][])  [unwired: 2 out]
        n3699 = shared-variable ".\\Zeiss Library.lvlib\\Det B Img"() -> (w2785:i16[][])  [unwired: 2 out]
        n3700 = shared-variable ".\\Zeiss Library.lvlib\\FIB Img"() -> (w2774:i16[][])  [unwired: 1 in, 1 out]
        n3701 = local read "SEM Scan Parameters"() -> (w2627:T26)
        n3702 = local read "Alert Settings"() -> (w2636:T36)
        n3703 = local read "SEM shutter status"() -> (w2630:string)
        n3704 = local read "SEM-FIB Delay (s)"() -> (w2621:u32)
        n3705 = shared-variable ".\\Zeiss Library.lvlib\\Tiled Image fit to"("Tiled Image fit to") -> ()  [unwired: 1 in, 1 out]
        n3706 = Wait Until Next ms Multiple(millisecond multiple=u32 100) -> ()  [unwired: 1 out]
        n3707 = Variant To Data(type=w2808, Variant=w2816) -> (data=w2807:T12)  [unwired: 1 in, 1 out]
        n3708 = Equal?(x=w2816, y=w2815) -> (x = y?=w2811:bool)
        n3709 = local read "Status message"() -> (w2699:string)
        n3710 = Unbundle By Name(w2636) -> ("Focus index low limit"=w2637:sgl, "Focus index stop limit"=w2638:sgl)
        n3711 = Equal?(x=w2792, y=w2791) -> (x = y?=w2790:bool[][])
        n3712 = Equal?(x=w2784, y=w2785) -> (x = y?=w2789:bool[][])
        n3713 = Equal?(x=w2777, y=w2774) -> (x = y?=w2776:bool[][])
        n3714 = Unbundle By Name(w2627) -> ("Frames"=w2629:u8, "Scan rate (Hz)"=w2826:u32, "X size (um)"=w2715:sgl, "Y size (um)"=w2712:sgl, "Frame line rampdown ratio"=w2827:sgl, "Pixel size (nm)"=w2642:sgl)
        n3715 = Unbundle By Name(w2627) -> ("X tiles"=w2625:u8, "Y tiles"=w2624:u8)
        n3716 = case shown="\"Unknown\", Default" w2630 {
          tunnel: [u32 16776960 u32 6618880 u32 16711680] -> w2631
          frame "Unknown", Default {
          }
          frame "Open" {
          }
          frame "Closed" {
          }
        }
        n3717 = Greater Than 0?(x=w2621) -> (x > 0?=w2620:bool)
        n3718 = And Array Elements(Boolean array=w2790) -> (logical AND=w2788:bool)
        n3719 = And Array Elements(Boolean array=w2789) -> (logical AND=w2787:bool)
        n3720 = And Array Elements(Boolean array=w2776) -> (logical AND=w2775:bool)
        n3721 = Unbundle By Name(w2807) -> ("Remaining time (m)"=w2814:u16, "Remaining time (s)"=w2813:u8)
        n3722 = And(x=w2788, y=w2787) -> (x .and. y?=w2786:bool)
        n3723 = property on="After SEM" class="Bool (strict)"("Visible"=w2620) -> ()  [unwired: 2 in, 2 out]
        n3724 = Unbundle By Name("FIB Options") -> ("Det"=w2802:u16)
        n3725 = property on="SEM shutter status" class="Str"("Text.BGColor"=w2631) -> ()  [unwired: 2 in, 2 out]
        n3726 = expression code="x/1000"(w2642) -> (w2711:sgl)
        n3727 = Multiply(x=w2625, y=w2624) -> (x*y=w2623:u8)
        n3728 = case shown="False" w2786 {
          tunnel: w2791 -> [w3071 _]
          tunnel: w2785 -> [w3070 _]
